vi "Write Status Updated Msg.vi"(10 "Chat Window UI Controller.lvlib:Status Updated Msg.lvclass":refnum<class "Status Updated Msg.lvclass">, 11 "Chat Window UI Controller in":refnum<class "Chat Window UI Controller.lvclass">) -> (3 "Chat Window UI Controller out":refnum<class "Chat Window UI Controller.lvclass">)   [LabVIEW 2015, in "Chat Window UI Controller.lvlib" / "Chat Window UI Controller.lvclass"]
uses:
  Chat Window UI Controller.lvclass
  Chat Window UI Controller Messages/Status Updated Msg/Status Updated Msg.lvclass
  Chat Window UI Controller.lvclass/Chat Window UI Controller.ctl
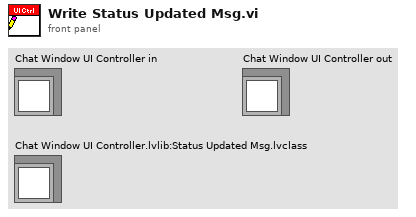
[diagram p1: front panel]
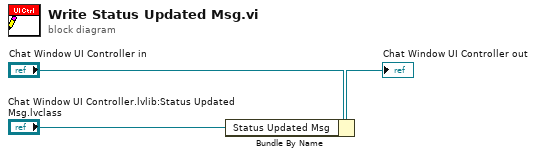
[diagram p0: block diagram]
diagram:
  n1 = Bundle By Name(cluster="Chat Window UI Controller in", "Status Updated Msg"="Chat Window UI Controller.lvlib:Status Updated Msg.lvclass") -> (→"Chat Window UI Controller out":refnum<class "Chat Window UI Controller.lvclass">)
